vi "oscSetup.vi"(2 "error in":errorcluster caption="Error in" {"code" format="%.0x"}, 3 "resource name 5112":refnum<k15>, 4 "Oscilloscope Setting Information String":string) -> (0 "error out":errorcluster caption="Error out" {"code" format="%.0x"}, 1 "output cluster":T1={"instrument handle out"="", "remaining string"="", "Settings"={"Horizontal Conf."={"Min. Sample rate"=0.0, "Reference position"=0.0, "Record Length"=0}, "Channel A"={"Enable"=FALSE, "Vertical coupling"=0.0, "Vertical range"=0.0, "Vertical offset"=0.0, "Probe attenuation"=1.0}, "Channel B"={"Enable"=FALSE, "Vertical coupling"=0.0, "Vertical range"=0.0, "Vertical offset"=0.0, "Probe attenuation"=1.0}, "Trigger"={"Source"=enum."channel 1", "Slope"=enum."Positive", "Coupling"=enum."AC", "Level"=0.0, "Holdoff"=0.0, "Delay"=0.0, " Timeout"=0.0, " Mode"=enum."Normal"}, "Measurements"={"Measurement 1, Channel"=enum."Channel 1", "Measurement 1, Selection"=0, "Measurement 2, Channel"=enum."Channel 1", "Measurement 2,  Selection"=0, "Measurement 3, Channel"=enum."Channel 1", "Measurement 3, Selection 3"=0}}})   [LabVIEW 2011]
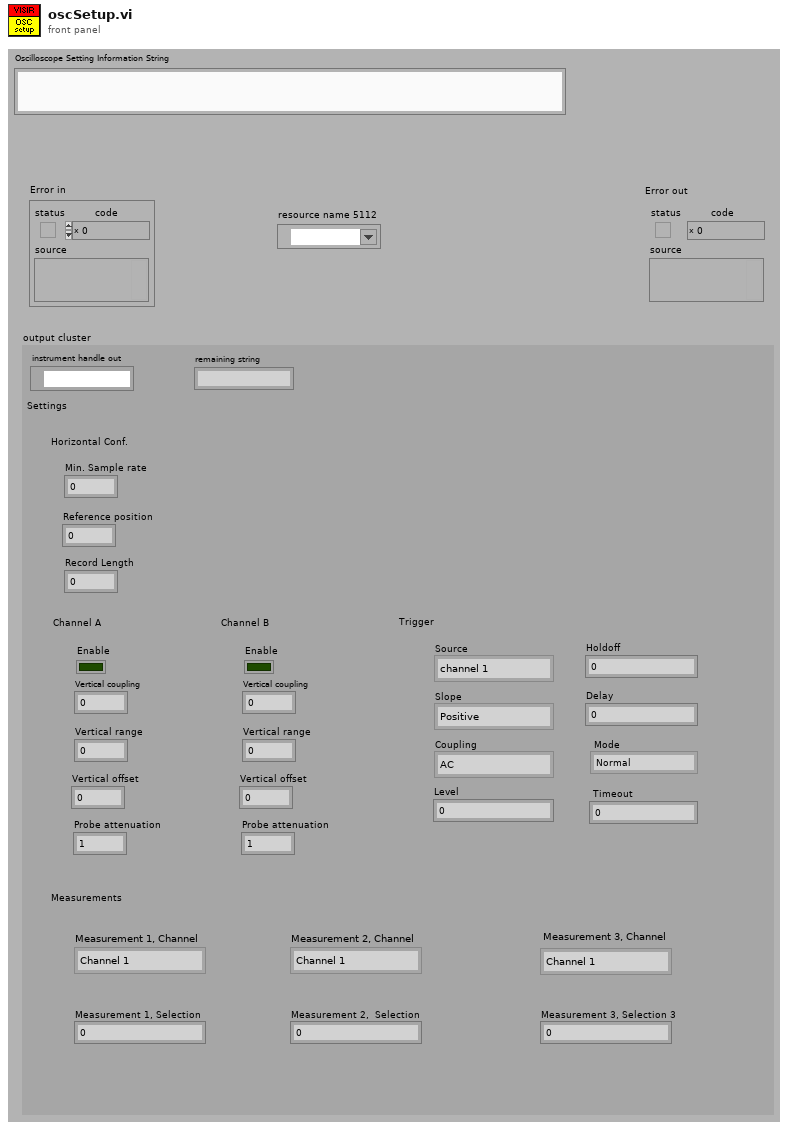
[diagram p1: front panel]
types:
  T1 = cluster{"instrument handle out":refnum<k15>, "remaining string":string, "Settings":cluster{"Horizontal Conf.":cluster{"Min. Sample rate":dbl, "Reference position":dbl, "Record Length":i16}, "Channel A":cluster{"Enable":bool, "Vertical coupling":dbl, "Vertical range":dbl, "Vertical offset":dbl, "Probe attenuation":dbl}, "Channel B":cluster{"Enable":bool, "Vertical coupling":dbl, "Vertical range":dbl, "Vertical offset":dbl, "Probe attenuation":dbl}, "Trigger":cluster{"Source":enum8{"channel 1", "channel 2", "Imediate", "External trigger"}, "Slope":enum8{"Positive", "Negative"}, "Coupling":enum8{"AC", "DC"}, "Level":dbl, "Holdoff":dbl, "Delay":dbl, " Timeout":dbl, " Mode":enum8{"Normal", "Auto", "Auto Level"}}, "Measurements":cluster{"Measurement 1, Channel":enum8{"Channel 1", "Channel 2", "Channel 3", "Channel 4"}, "Measurement 1, Selection":u16, "Measurement 2, Channel":enum8{"Channel 1", "Channel 2", "Channel 3", "Channel 4"}, "Measurement 2,  Selection":u16, "Measurement 3, Channel":enum8{"Channel 1", "Channel 2", "Channel 3", "Channel 4"}, "Measurement 3, Selection 3":u16}}}
  T2 = cluster{"Horizontal Conf.":cluster{"Min. Sample rate":dbl, "Reference position":dbl, "Record Length":i16}, "Channel A":cluster{"Enable":bool, "Vertical coupling":i32, "Vertical range":dbl, "Vertical offset":dbl, "Probe attenuation":dbl}, "Channel B":cluster{"Enable":bool, "Vertical coupling":i32, "Vertical range":dbl, "Vertical offset":dbl, "Probe attenuation":dbl}, "Trigger":cluster{"Source":enum8{"channel 1", "channel 2", "Imediate", "External trigger"}, "Slope":enum8{"Positive", "Negative"}, "Coupling":enum8{"AC", "DC"}, "Level":dbl, "Holdoff":dbl, "Delay":dbl, " Timeout":dbl, " Mode":enum8{"Normal", "Auto", "Auto Level", ""}}, "Measurements":cluster{"Measurement 1, Channel":enum8{"Channel 1", "Channel 2", "Channel 3", "Channel 4"}, "Measurement 1, Selection":u16, "Measurement 2, Channel":enum8{"Channel 1", "Channel 2", "Channel 3", "Channel 4"}, "Measurement 2,  Selection":u16, "Measurement 3, Channel":enum8{"Channel 1", "Channel 2", "Channel 3", "Channel 4"}, "Measurement 3, Selection 3":u16}}
  T3 = cluster{"instrument handle out":refnum<k15>, "Remaining string":string, "Settings":cluster{"Horizontal Conf.":cluster{"Min. Sample rate":dbl, "Reference position":dbl, "Record Length":i16}, "Channel A":cluster{"Enable":bool, "Vertical coupling":i32, "Vertical range":dbl, "Vertical offset":dbl, "Probe attenuation":dbl}, "Channel B":cluster{"Enable":bool, "Vertical coupling":i32, "Vertical range":dbl, "Vertical offset":dbl, "Probe attenuation":dbl}, "Trigger":cluster{"Source":enum8{"channel 1", "channel 2", "Imediate", "External trigger"}, "Slope":enum8{"Positive", "Negative"}, "Coupling":enum8{"AC", "DC"}, "Level":dbl, "Holdoff":dbl, "Delay":dbl, " Timeout":dbl, " Mode":enum8{"Normal", "Auto", "Auto Level", ""}}, "Measurements":cluster{"Measurement 1, Channel":enum8{"Channel 1", "Channel 2", "Channel 3", "Channel 4"}, "Measurement 1, Selection":u16, "Measurement 2, Channel":enum8{"Channel 1", "Channel 2", "Channel 3", "Channel 4"}, "Measurement 2,  Selection":u16, "Measurement 3, Channel":enum8{"Channel 1", "Channel 2", "Channel 3", "Channel 4"}, "Measurement 3, Selection 3":u16}}}
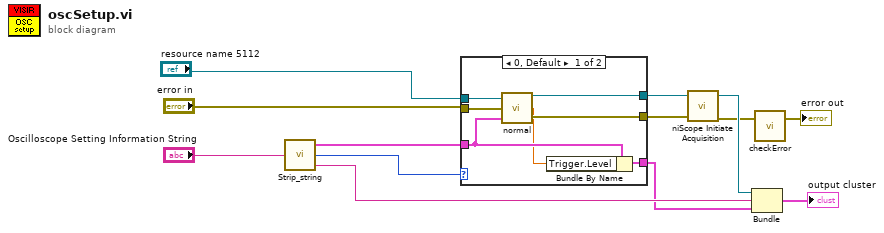
[diagram p0: block diagram]
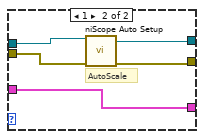
[diagram p2: hidden frame]
diagram:
  n1 = call "Strip_string.vi"("Oscilloscope Setting Information Normal mode"="Oscilloscope Setting Information String") -> ("Settings"=w5:T2, "Autoscale?"=w7:i8, "Remaining string"=w10:string)
  n2 = case shown="0, Default" w7 {
    tunnel: [w18 w21] -> w13
    tunnel: [w19 w22] -> w12
    tunnel: "resource name 5112" -> [w14 w24]
    tunnel: "error in" -> [w20 w23]
    tunnel: w5 -> [w17 w25]
    tunnel: [w15 w25] -> w6
    frame 0, Default {
      n3 = call "normal.vi"("Settings"=w17, "error in"=w20, "instrument handle in"=w14) -> ("error out"=w18:errorcluster, "Adjusted Trigger Level"=w16:dbl, "instrument handle out"=w19:refnum<k15>)
      n4 = Bundle By Name(cluster=w17, "Trigger.Level"=w16) -> (w15:T2)
    }
    frame 1 {
      # "AutoScale"
      n5 = call <instrlib>:"niScope Auto Setup.vi"("instrument handle"=w24, "error in"=w23) -> ("instrument handle out"=w22:refnum<k15>, "error out"=w21:errorcluster)  [unwired: 12 in]
    }
  }
  n6 = call <instrlib>:"niScope Initiate Acquisition.vi"("instrument handle"=w12, "error in"=w13) -> ("instrument handle out"=w11:refnum<k15>, "error out"=w2:errorcluster)  [unwired: 12 in]
  n7 = Bundle("instrument handle out"=w11, "Remaining string"=w10, "Settings"=w6) -> (→"output cluster":T3)  [unwired: 1 in]
  n8 = call "checkError.vi"("error in"=w2) -> ("error out"=→"error out":errorcluster)  [unwired: 1 in, 1 out]
